vi "Wait_ms.vi"(6 "等待时间（毫秒）":u32=100, 8 "错误输入（无错误）":errorcluster) -> (0 "error IO":errorcluster)   [LabVIEW 2012]
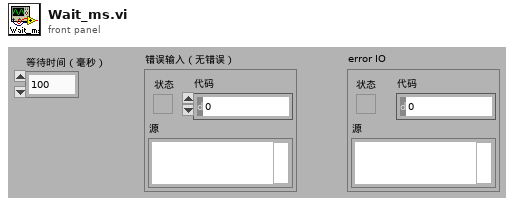
[diagram p1: front panel]
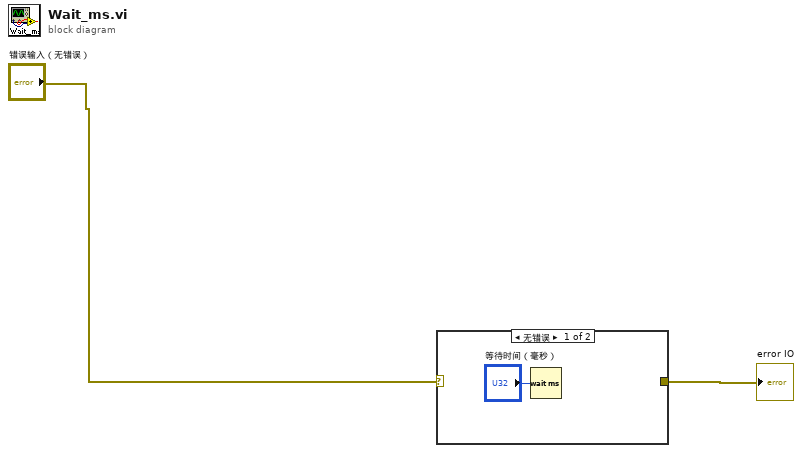
[diagram p0: block diagram]
diagram:
  n1 = case shown="无错误" "错误输入（无错误）" {
    selector: "错误输入（无错误）" -> [_ w4]
    tunnel: [_ w4] -> w2
    frame No Error {
      n2 = Wait (ms)(milliseconds to wait="等待时间（毫秒）") -> ()  [unwired: 1 out]
    }
    frame Error {
    }
  }
  "error IO" <- w2
